vi "PathPlanner_FindPath.vi"() -> ()   [LabVIEW 2019]
uses:
  <vilib>/Rock Robotics/WPI/ThirdParty/JAS_Junk/TrajLib/TypeDef/TRANSLATION2D.ctl
  <vilib>/Rock Robotics/WPI/ThirdParty/MJansen/PathPlanner/TypeDef/PathPlannerGoalEndState.ctl
  <vilib>/Rock Robotics/WPI/ThirdParty/JAS_Junk/TrajLib/TypeDef/ROTATION2D.ctl
  <vilib>/Rock Robotics/WPI/ThirdParty/MJansen/PathPlanner/TypeDef/PathPlannerPath.ctl
  <vilib>/Rock Robotics/WPI/ThirdParty/MJansen/PathPlanner/TypeDef/PathPlannerRotationTarget.ctl
  <vilib>/Rock Robotics/WPI/ThirdParty/MJansen/PathPlanner/TypeDef/PathPlannerConstraintsZone.ctl
  <vilib>/Rock Robotics/WPI/ThirdParty/MJansen/PathPlanner/TypeDef/PathPlannerPathConstraints.ctl
  <vilib>/Rock Robotics/WPI/ThirdParty/MJansen/PathPlanner/TypeDef/PathPlannerEventMarker.ctl
  <vilib>/Rock Robotics/WPI/ThirdParty/MJansen/PathPlanner/TypeDef/PathPlannerCommandUtil.ctl
  <vilib>/Rock Robotics/WPI/ThirdParty/MJansen/PathPlanner/ENum/PathPlanner_CommandUtilType_ENUM.ctl
  <vilib>/Rock Robotics/WPI/ThirdParty/MJansen/PathPlanner/TypeDef/PathPlannerPathPoint.ctl
  <vilib>/Rock Robotics/WPI/ThirdParty/JAS_Junk/TrajLib/TypeDef/CHASSIS_SPEEDS.ctl
  <vilib>/Rock Robotics/WPI/ThirdParty/MJansen/PathPlanner/VI/PathPlanner_GridPosition_Get.vi
  <vilib>/Rock Robotics/WPI/ThirdParty/JAS_Junk/TrajLib/Translation2d_Create.vi
  <vilib>/Rock Robotics/WPI/ThirdParty/MJansen/PathPlanner/VI/PathPlanner_PathFinder_Globals.vi
  <vilib>/robotics/Navigation/shared/WorldMap/OccupancyGridWorldMap/NI_Robotics_OccupancyGridWorldMap.lvclass
  <vilib>/robotics/Navigation/shared/MapNode/AbstractDstarNode/NI_Robotics_AbstractDstarNode.lvclass
  <vilib>/Rock Robotics/WPI/ThirdParty/MJansen/PathPlanner/PathPlanner24.lvlib
  <vilib>/Rock Robotics/WPI/ThirdParty/JAS_Junk/TrajLib/Trajectory_Library.lvlib
panel:
  out "Extract Simplified Path Size":i32
  out "Do Reset Err Count":i64
  out "Do Minor Err Count":i64
  out "Do Major Err Count":i64
  out "Extract Path Size":i32
  out "Field":cluster{dbl[], dbl[]}[](graph)
  out "Error_No_Path":bool
  out "New Path Available":bool
  out "Loop Count":i32
  out "Do Work Count":i64
  out "Do Reset Count":i64
  out "Do Minor Count":i64
  out "Do Major Count":i64
  out "PathPlannerPath":T1={"BezierPoints"=[], "PreviewStartingRotation"={"VALUE"=0.0, "COS"=1.0, "SIN"=0.0}, "Reversed"=FALSE, "RotationTargets"=[], "ConstraintZones"=[], "EventMarkers"=[], "GlobalConstraints"={"MaxVelocityMps;"=0.0, "MaxAccelerationMpsSq;"=0.0, "MaxAngularVelRadPsEc;"=0.0, "MaxAngularAccRadPSecSq"=0.0, "Exists"=FALSE}, "GoalEndState"={"Velocity"=0.0, "Rotation"={"VALUE"=0.0, "COS"=1.0, "SIN"=0.0}}, "AllPoints"=[]} {"AllPoints"."HolonomicRotation"."SIN" format="%13.4f"; "AllPoints"."HolonomicRotation"."COS" format="%13.4f"; "AllPoints"."HolonomicRotation"."VALUE" format="%13.4f"; "AllPoints"."Position"."Y" format="%14.3f"; "AllPoints"."Position"."X" format="%14.3f"; "GoalEndState"."Rotation"."SIN" format="%13.4f"; "GoalEndState"."Rotation"."COS" format="%13.4f"; "GoalEndState"."Rotation"."VALUE" format="%13.4f"; "EventMarkers"."lastRobotPos"."Y" format="%14.3f"; "EventMarkers"."lastRobotPos"."X" format="%14.3f"; "EventMarkers"."markerPos"."Y" format="%14.3f"; "EventMarkers"."markerPos"."X" format="%14.3f"; "RotationTargets"."target"."SIN" format="%13.4f"; "RotationTargets"."target"."COS" format="%13.4f"; "RotationTargets"."target"."VALUE" format="%13.4f"; "PreviewStartingRotation"."SIN" format="%13.4f"; "PreviewStartingRotation"."COS" format="%13.4f"; "PreviewStartingRotation"."VALUE" format="%13.4f"; "BezierPoints"."Y" format="%14.3f"; "BezierPoints"."X" format="%14.3f"}
  in  "GoalEndState":T10={"Velocity"=0.0, "Rotation"={"VALUE"=0.0, "COS"=1.0, "SIN"=0.0}} {"Rotation"."SIN" format="%13.4f"; "Rotation"."COS" format="%13.4f"; "Rotation"."VALUE" format="%13.4f"}
  in  "Goal Position":T2={"X"=14.0, "Y"=6.5} {"Y" step=0.25 format="%14.3f"; "X" step=0.25 format="%14.3f"}
  in  "StartPosition":T2={"X"=1.5, "Y"=1.5} {"Y" step=0.25 format="%14.3f"; "X" step=0.25 format="%14.3f"}
  out "NewPathAvailLastCheck":i32
  out "NewPathAvailCount":i32
  out "BackGroundInitialized":bool
  # "Before running, copy the files from the DEPLOY directory to the <user>\\Documents\\LabVIEW Data directory."
  # "Change Starting \nand Goal (target)\nPositions to update\npath."
  # "These values are\nonly for debugging"
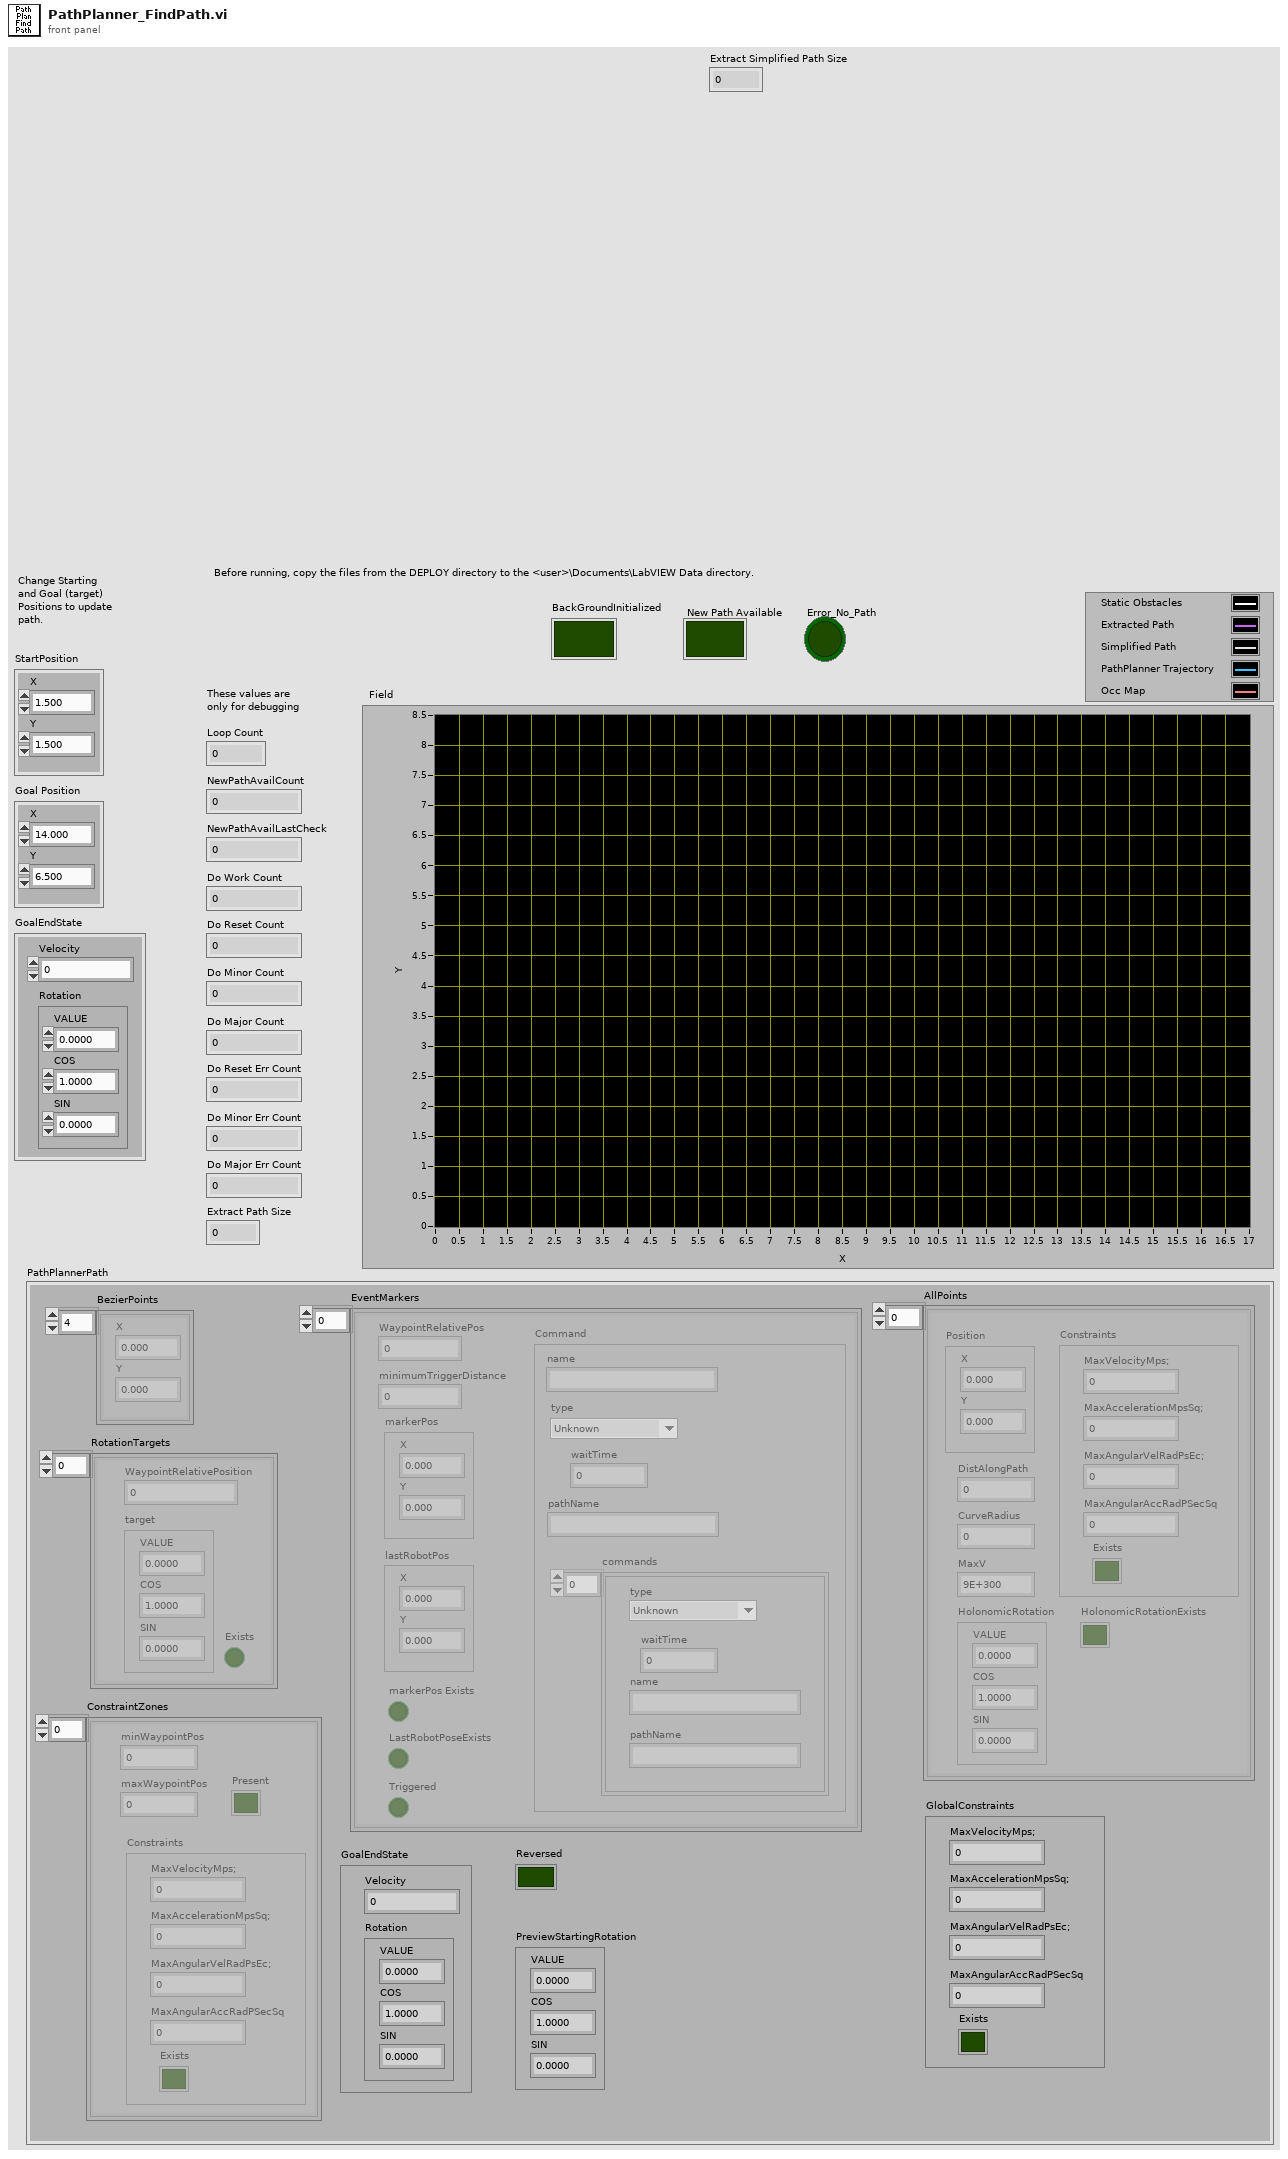
[diagram p1: front panel]
types:
  T1 = typedef "PathPlanner24.lvlib/PathPlannerPath.ctl" = cluster{"BezierPoints":T2[], "PreviewStartingRotation":T3, "Reversed":bool, "RotationTargets":T4[], "ConstraintZones":T5[], "EventMarkers":T7[], "GlobalConstraints":T6, "GoalEndState":T10, "AllPoints":T11[]}
  T2 = typedef "Trajectory_Library.lvlib/TRANSLATION2D.ctl" = cluster{"X":dbl, "Y":dbl}
  T3 = typedef "Trajectory_Library.lvlib/ROTATION2D.ctl" = cluster{"VALUE":dbl, "COS":dbl, "SIN":dbl}
  T4 = typedef "PathPlanner24.lvlib/PathPlannerRotationTarget.ctl" = cluster{"target":T3, "WaypointRelativePosition":dbl, "Exists":bool}
  T5 = typedef "PathPlanner24.lvlib/PathPlannerConstraintsZone.ctl" = cluster{"minWaypointPos":dbl, "maxWaypointPos":dbl, "Constraints":T6, "Present":bool}
  T6 = typedef "PathPlanner24.lvlib/PathPlannerPathConstraints.ctl" = cluster{"MaxVelocityMps;":dbl, "MaxAccelerationMpsSq;":dbl, "MaxAngularVelRadPsEc;":dbl, "MaxAngularAccRadPSecSq":dbl, "Exists":bool}
  T7 = typedef "PathPlanner24.lvlib/PathPlannerEventMarker.ctl" = cluster{"WaypointRelativePos":dbl, "minimumTriggerDistance":dbl, "markerPos":T2, "lastRobotPos":T2, "Command":T8, "markerPos Exists":bool, "LastRobotPoseExists":bool, "Triggered":bool}
  T8 = typedef "PathPlanner24.lvlib/PathPlannerCommandUtil.ctl" = cluster{"waitTime":dbl, "name":string, "pathName":string, "commands":cluster{"type":T9, "waitTime":dbl, "name":string, "pathName":string}[], "type":T9}
  T9 = typedef "PathPlanner24.lvlib/PathPlanner_CommandUtilType_ENUM.ctl" = enum16{"Unknown", "Wait", "Named", "Path", "Sequential", "Parallel", "Race", "Deadline"}
  T10 = typedef "PathPlanner24.lvlib/PathPlannerGoalEndState.ctl" = cluster{"Velocity":dbl, "Rotation":T3}
  T11 = typedef "PathPlanner24.lvlib/PathPlannerPathPoint.ctl" = cluster{"Position":T2, "HolonomicRotation":T3, "DistAlongPath":dbl, "CurveRadius":dbl, "MaxV":dbl, "Constraints":T6, "HolonomicRotationExists":bool}
  T12 = typedef "Trajectory_Library.lvlib/CHASSIS_SPEEDS.ctl" = cluster{"vX":dbl, "vY":dbl, "vOmega":dbl}
  T13 = cluster{"DoResetErrCount":i64, "DoResetCount":i64, "DoMinorErrCount":i64, "DoMinorCount":i64, "DoMajorErrCount":i64, "DoMajorCount":i64, "DoWorkLoopCount":i64, "BackGroundInitialized":bool, "TerminateWorker":bool}
  T14 = typedef "PathPlanner24.lvlib/PathPlannerFinderGridPosition.ctl" = cluster{"X":i32, "Y":i32}
  T15 = cluster{"ExtractedPath":T14[], "ExtractedPathSimplified":T14[], "ExtractedFieldPosPath":T2[], "CurrentPath":T2[], "Obstacles":set{T14}, "StaticOccupancyGrid":refnum<data-value>, "path references":refnum<data-value>[], "Main Program Name":string}
  T16 = typedef "PathPlanner24.lvlib/PathPlannerTrajectory.ctl" = cluster{"States":T17[]}
  T17 = typedef "PathPlanner24.lvlib/PathPlannerTrajectoryState.ctl" = cluster{"TimeSeconds":dbl, "VelocityMPS":dbl, "AccerationMpsSq":dbl, "HeadingAngularVelRadPerSec":dbl, "PositionMeters":T2, "Heading":T3, "TargetHolonomicRotation":T3, "CurvatureRadPerMeter":dbl, "PathPlannerConstraints":T6, "DeltaPos":dbl}
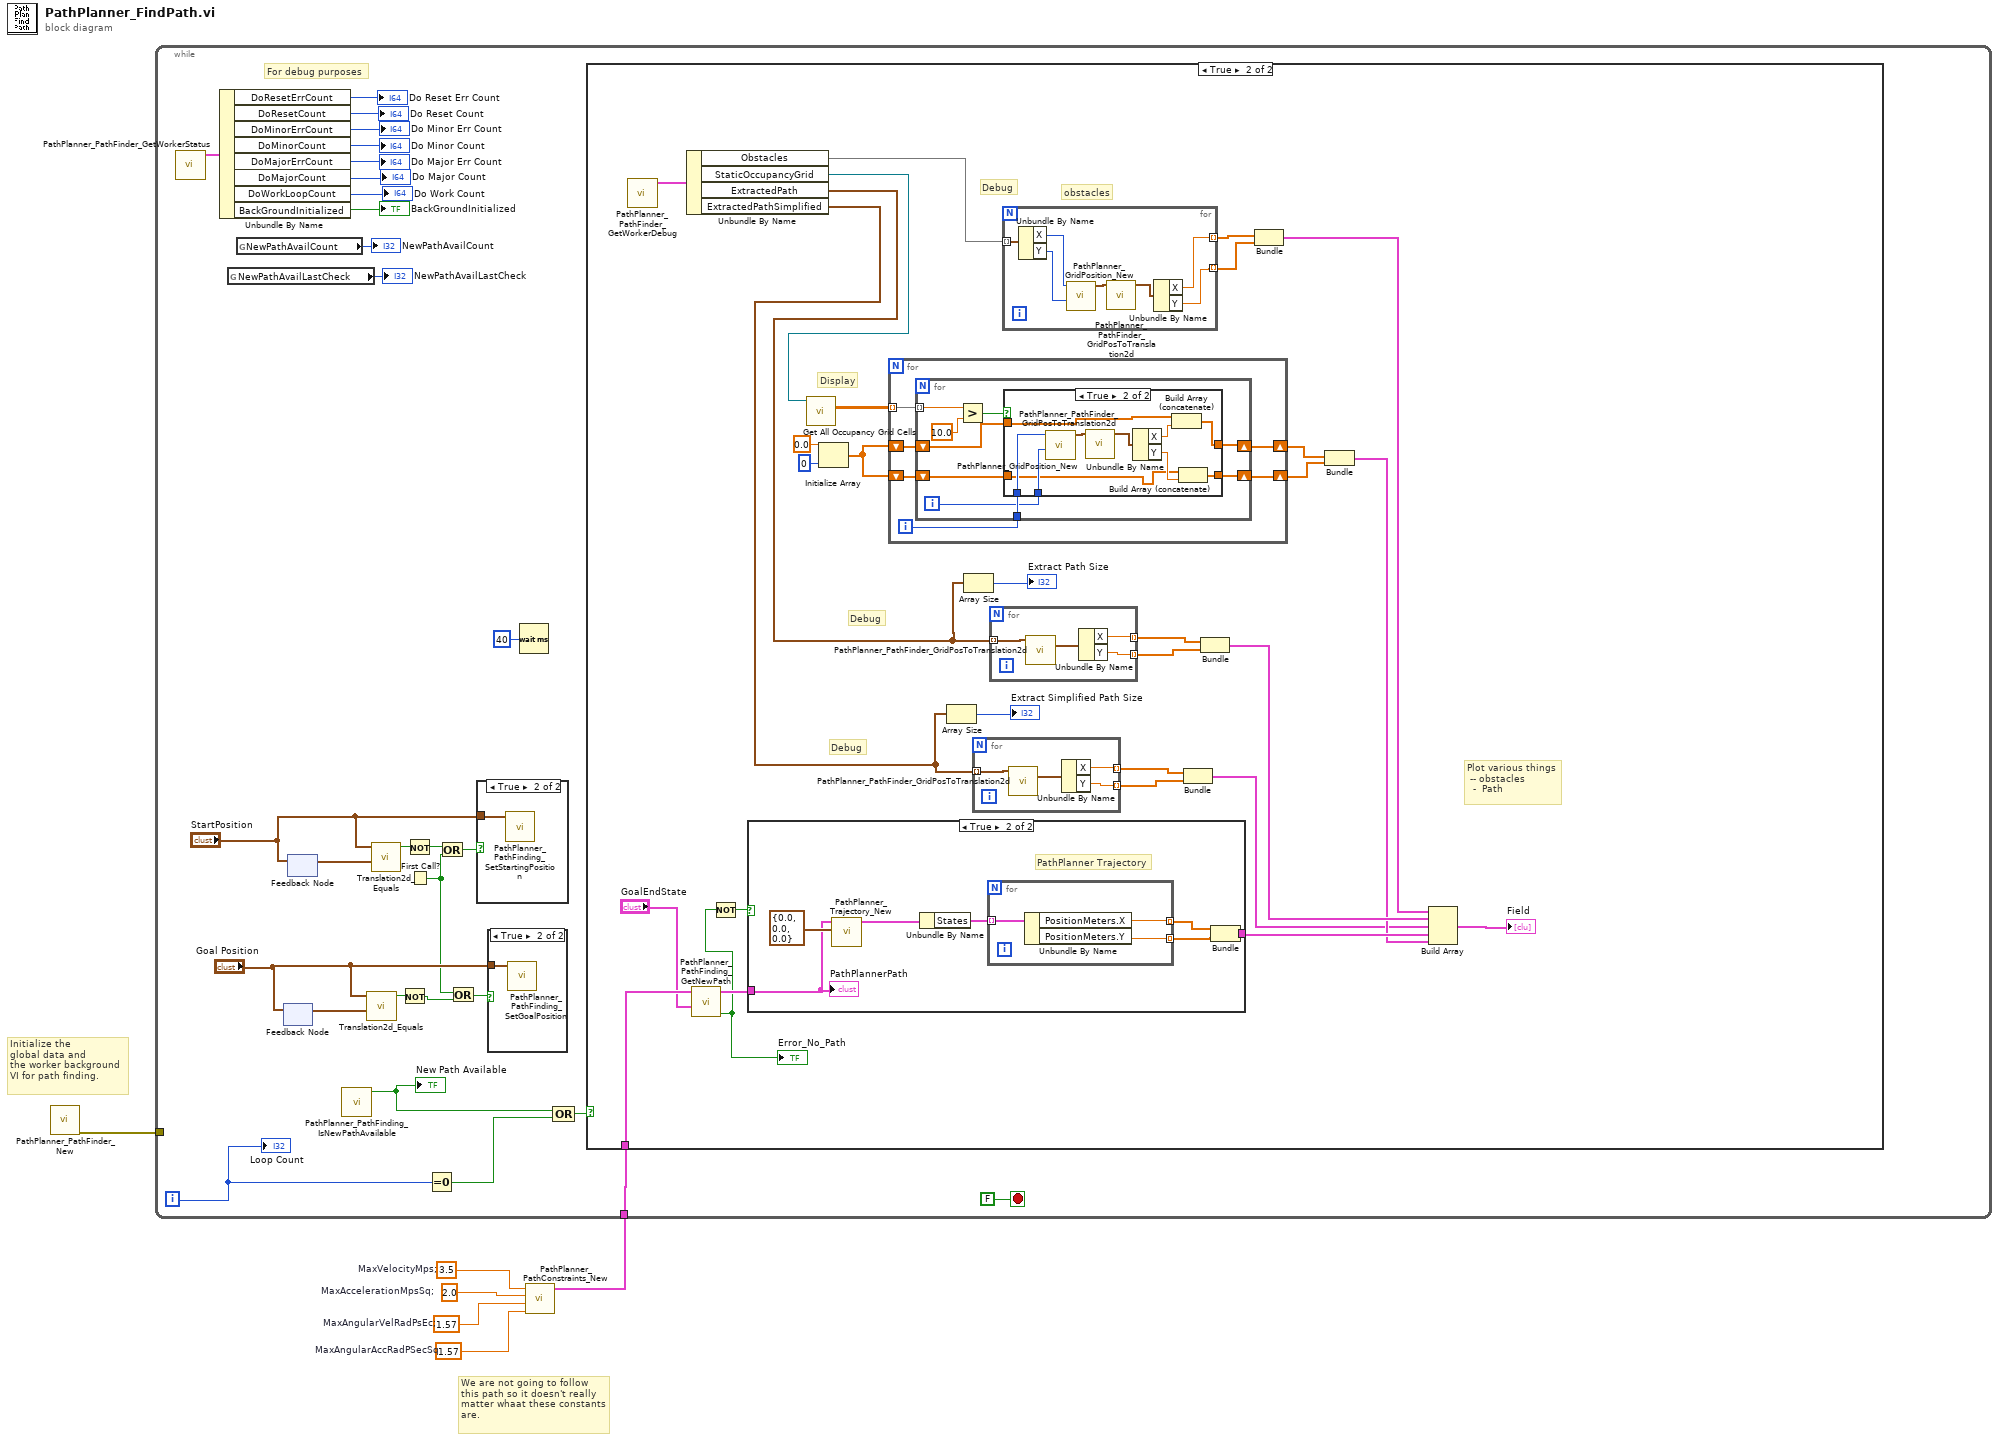
[diagram p0: block diagram]
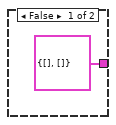
[diagram p3: hidden frame]
diagram:
  w2 = 3.5  # MaxVelocityMps;
  w3 = 2.0  # MaxAccelerationMpsSq;
  w4 = 1.57  # MaxAngularVelRadPsEc;
  w5 = 1.57  # MaxAngularAccRadPSecSq
  # "We are not going to follow\nthis path so it doesn't really\nmatter whaat these constants\nare."
  # "Initialize the \nglobal data and\nthe worker background\nVI for path finding."
  n1 = call <vilib>:"PathPlanner_PathFinder_New.vi"() -> ("error out"=w1:errorcluster)  [unwired: 11 in]
  n2 = call <vilib>:"PathPlanner_PathConstraints_New.vi"("MaxAngularAccRadPSecSq"=w5, "MaxAngularVelRadPsEc;"=w4, "MaxAccelerationMpsSq;"=w3, "MaxVelocityMps;"=w2) -> ("PathPlannerConstraints"=w6:T6)  [unwired: 7 in]
  n3 = while {
    tunnel: w6 -> [w28]
    tunnel: w1 -> [_]
    i -> [w30]
    stop <- FALSE stop-if-true
    # "For debug purposes"
    n4 = call <vilib>:"PathPlanner_PathFinder_GetWorkerStatus.vi"() -> ("PathFindingWorkerStatus"=w15:T13)  [unwired: 11 in]
    n5 = Unbundle By Name(w15) -> ("DoResetErrCount"=→"Do Reset Err Count":i64, "DoResetCount"=→"Do Reset Count":i64, "DoMinorErrCount"=→"Do Minor Err Count":i64, "DoMinorCount"=→"Do Minor Count":i64, "DoMajorErrCount"=→"Do Major Err Count":i64, "DoMajorCount"=→"Do Major Count":i64, "DoWorkLoopCount"=→"Do Work Count":i64, "BackGroundInitialized"=→"BackGroundInitialized":bool)
    n6 = global read "PathPlanner_PathFinder_Globals.vi" "NewPathAvailLastCheck"() -> (→"NewPathAvailLastCheck":i32)
    n7 = global read "PathPlanner_PathFinder_Globals.vi" "NewPathAvailCount"() -> (→"NewPathAvailCount":i32)
    n8 = feedback #1() -> (w32:T2)  [unwired: 1 in]
    n9 = feedback-in #1("Goal Position") -> ()
    n10 = feedback-in #2("StartPosition") -> ()
    n11 = feedback #2() -> (w34:T2)  [unwired: 1 in]
    n12 = call <vilib>:"PathPlanner_PathFinding_IsNewPathAvailable.vi"() -> ("New Path Available"=w25:bool)  [unwired: 10 in, 1 out]
    "New Path Available" <- w25
    n13 = call <vilib>:"Translation2d_Equals.vi"("other Translation"=w32, "In Translation"="Goal Position") -> ("Equals"=w31:bool)  [unwired: 9 in]
    n14 = call <vilib>:"Translation2d_Equals.vi"("other Translation"=w34, "In Translation"="StartPosition") -> ("Equals"=w33:bool)  [unwired: 9 in]
    n15 = Not(x=w31) -> (.not. x?=w20:bool)
    n16 = Not(x=w33) -> (.not. x?=w18:bool)
    n17 = First Call?() -> (First Call?: T/F=w19:bool)
    n18 = Equal To 0?(x=w30) -> (x = 0?=w27:bool)
    n19 = Or(x=w18, y=w19) -> (x .or. y?=w22:bool)
    n20 = Or(x=w19, y=w20) -> (x .or. y?=w21:bool)
    n21 = case shown="True" w22 {
      tunnel: "StartPosition" -> [_ w120]
      frame False {
      }
      frame True {
        n22 = call <vilib>:"PathPlanner_PathFinding_SetStartingPosition.vi"("StartPosition"=w120) -> ()  [unwired: 10 in, 1 out]
      }
    }
    n23 = case shown="True" w21 {
      tunnel: "Goal Position" -> [_ w119]
      frame False {
      }
      frame True {
        n24 = call <vilib>:"PathPlanner_PathFinding_SetGoalPosition.vi"("GoalPosition"=w119) -> ()  [unwired: 10 in, 1 out]
      }
    }
    n25 = Wait (ms)(milliseconds to wait=u32 40) -> ()  [unwired: 1 out]
    n26 = Compound Arithmetic op=OR(w25, w27) -> (w29:bool)
    n27 = case shown="True" w29 {
      tunnel: w28 -> [_ w60]
      frame False {
      }
      frame True {
        # "Plot various things\n -- obstacles\n  -  Path"
        # "Debug"
        # "Display"
        # "Debug"
        # "Debug"
        # "obstacles"
        n28 = call <vilib>:"PathPlanner_PathFinder_GetWorkerDebug.vi"() -> ("PathFinderWorkerDebug"=w42:T15)  [unwired: 11 in]
        n29 = Unbundle By Name(w42) -> ("Obstacles"=w41:set{T14}, "StaticOccupancyGrid"=w40:refnum<data-value>, "ExtractedPath"=w39:T14[], "ExtractedPathSimplified"=w38:T14[])
        n30 = call <vilib>:"PathPlanner_PathFinding_GetNewPath.vi"("GoalEndState"="GoalEndState", "PathPlannerPathConstraints"=w60) -> ("Error_No_Path"=w36:bool, "PathPlannerPath"=w58:T1)  [unwired: 8 in]
        "Error_No_Path" <- w36
        n31 = Not(x=w36) -> (.not. x?=w37:bool)
        n32 = case shown="True" w37 {
          tunnel: w58 -> [_ w71]
          tunnel: [cluster{dbl[], dbl[]} {[], []} w67] -> w55
          frame False {
          }
          frame True {
            # "PathPlanner Trajectory"
            n33 = call <vilib>:"PathPlanner_Trajectory_New.vi"("StartingSpeeds"=T12 {"vX"=0.0, "vY"=0.0, "vOmega"=0.0}, "Path"=w71) -> ("PathPlannerTrajectory"=w72:T16)  [unwired: 9 in]
            n34 = Unbundle By Name(w72) -> ("States"=w70:T17[])
            n35 = for {
              tunnel: [w75] -> w69 mode=indexing
              tunnel: [w76] -> w68 mode=indexing
              tunnel: w70 -> [w74] mode=indexing
              n36 = Unbundle By Name(w74) -> ("PositionMeters.X"=w75:dbl, "PositionMeters.Y"=w76:dbl)
            }
            n37 = Bundle(w69, w68) -> (w67:cluster{dbl[], dbl[]})  [unwired: 1 in]
            "PathPlannerPath" <- w71
          }
        }
        n38 = call <vilib>:"Get All Occupancy Grid Cells.vi"("map reference in"=w40) -> ("occupancy grid"=w46:dbl[][])  [unwired: 8 in, 2 out]
        n39 = Initialize Array(0.0 ("element"), 0 ("dimension size")) -> (w43:dbl[])
        n40 = for {
          tunnel: w46 -> [w86] mode=indexing
          shift-right: [w82] -> w53
          shift-left: w43 -> [w85]
          shift-right: [w81] -> w52
          shift-left: w43 -> [w84]
          i -> [w83]
          n41 = for {
            tunnel: w86 -> [w95] mode=indexing
            shift-right: [w89] -> w82
            shift-left: w85 -> [w90]
            shift-right: [w87] -> w81
            shift-left: w84 -> [w88]
            tunnel: w83 -> [w92]
            i -> [w91]
            n42 = Greater?(x=w95, y=10.0) -> (0:w93:bool)
            n43 = case shown="True" w93 {
              tunnel: w92 -> [_ w106]
              tunnel: w91 -> [_ w102]
              tunnel: w90 -> [w97 w101]
              tunnel: [w97 w100] -> w89
              tunnel: w88 -> [w96 w99]
              tunnel: [w96 w98] -> w87
              frame False {
              }
              frame True {
                n44 = call <vilib>:"PathPlanner_GridPosition_New.vi"("Int Y"=w102, "Int X"=w106) -> ("GridPosition"=w107:T14)  [unwired: 9 in]
                n45 = call <vilib>:"PathPlanner_PathFinder_GridPosToTranslation2d.vi"("GridPosition"=w107) -> ("RealGridPos"=w105:T2)  [unwired: 10 in]
                n46 = Unbundle By Name(w105) -> ("X"=w104:dbl, "Y"=w103:dbl)
                n47 = Build Array (concatenate)(w101, w104) -> (w100:dbl[])
                n48 = Build Array (concatenate)(w99, w103) -> (w98:dbl[])
              }
            }
          }
        }
        n49 = Array Size(array=w38) -> (size(s)=→"Extract Simplified Path Size":i32)
        n50 = Array Size(array=w39) -> (size(s)=→"Extract Path Size":i32)
        n51 = for {
          tunnel: [w78] -> w50 mode=indexing
          tunnel: [w80] -> w49 mode=indexing
          tunnel: w38 -> [w77] mode=indexing
          n52 = call <vilib>:"PathPlanner_PathFinder_GridPosToTranslation2d.vi"("GridPosition"=w77) -> ("RealGridPos"=w79:T2)  [unwired: 10 in]
          n53 = Unbundle By Name(w79) -> ("X"=w78:dbl, "Y"=w80:dbl)
        }
        n54 = for {
          tunnel: [w109] -> w57 mode=indexing
          tunnel: [w111] -> w56 mode=indexing
          tunnel: w39 -> [w108] mode=indexing
          n55 = call <vilib>:"PathPlanner_PathFinder_GridPosToTranslation2d.vi"("GridPosition"=w108) -> ("RealGridPos"=w110:T2)  [unwired: 10 in]
          n56 = Unbundle By Name(w110) -> ("X"=w109:dbl, "Y"=w111:dbl)
        }
        n57 = for {
          tunnel: w41 -> [w118] mode=indexing
          tunnel: [w113] -> w64 mode=indexing
          tunnel: [w112] -> w65 mode=indexing
          n58 = Unbundle By Name(w118) -> ("X"=w115:i32, "Y"=w114:i32)
          n59 = call <vilib>:"PathPlanner_GridPosition_New.vi"("Int Y"=w114, "Int X"=w115) -> ("GridPosition"=w117:T14)  [unwired: 9 in]
          n60 = call <vilib>:"PathPlanner_PathFinder_GridPosToTranslation2d.vi"("GridPosition"=w117) -> ("RealGridPos"=w116:T2)  [unwired: 10 in]
          n61 = Unbundle By Name(w116) -> ("X"=w113:dbl, "Y"=w112:dbl)
        }
        n62 = Bundle(w50, w49) -> (w47:cluster{dbl[], dbl[]})  [unwired: 1 in]
        n63 = Bundle(w57, w56) -> (w61:cluster{dbl[], dbl[]})  [unwired: 1 in]
        n64 = Bundle(w64, w65) -> (w62:cluster{dbl[], dbl[]})  [unwired: 1 in]
        n65 = Bundle(w53, w52) -> (w54:cluster{dbl[], dbl[]})  [unwired: 1 in]
        n66 = Build Array(w62, w61, w47, w55, w54) -> (→"Field":cluster{dbl[], dbl[]}[])
      }
    }
    "Loop Count" <- w30
  }
